vi "BME_DG_ResetCounters.vi"(7 "EventCounter(True)":bool=TRUE, 8 "error in (no error)":errorcluster, 9 "TileList(True)":bool=TRUE, 10 "ModuloCounter(True)":bool=TRUE, 11 "DG_Number":i32) -> (0 "error out":errorcluster, 3 "return code":i32)   [LabVIEW 2009, in "POLARIS BME DG.lvlib"]
uses:
  POLARIS BME DG.lvlib
  BME DLL/DelayGenerator.dll
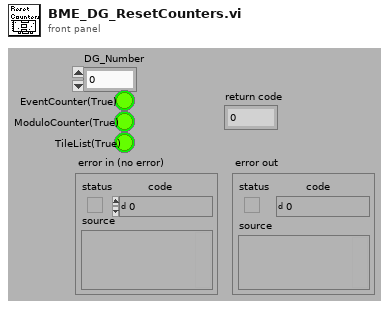
[diagram p1: front panel]
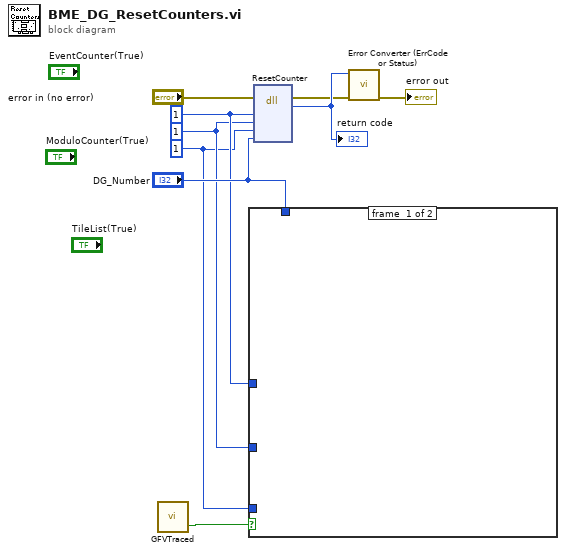
[diagram p0: block diagram]
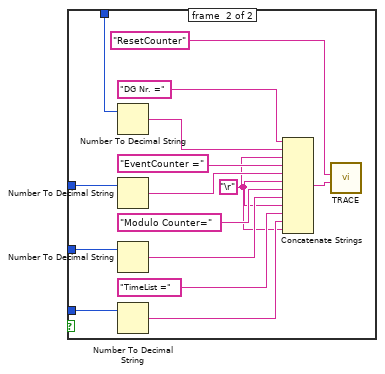
[diagram p2: hidden frame]
diagram:
  w1 = u32 1 ("bTimeList")
  w2 = u32 1 ("bTriggerCounter")
  w3 = u32 1 ("bEventCounter")
  n1 = call "GFVTraced.vi"() -> ("traced?"=w5:bool)  [unwired: 2 in]
  n2 = case shown="True" w5 {
    tunnel: w3 -> [_ w21]
    tunnel: w2 -> [_ w16]
    tunnel: "DG_Number" -> [_ w11]
    tunnel: w1 -> [_ w10]
    frame #0 {
    }
    frame #1 {
      w14 = "\r"
      n3 = Number To Decimal String(number=w11) -> (decimal integer string=w12:string)  [unwired: 1 in]
      n4 = Number To Decimal String(number=w21) -> (decimal integer string=w20:string)  [unwired: 1 in]
      n5 = Number To Decimal String(number=w16) -> (decimal integer string=w18:string)  [unwired: 1 in]
      n6 = Number To Decimal String(number=w10) -> (decimal integer string=w15:string)  [unwired: 1 in]
      n7 = Concatenate Strings("DG Nr. =", w12, w14, "EventCounter =", w20, w14, "Modulo Counter=", w18, w14, "TimeList =", w15, w14) -> (w22:string)
      n8 = call "TRACE.vi"("Parameter String"=w22, "Function"="ResetCounter") -> ()  [unwired: 10 in]
    }
  }
  n9 = dll-call lib="D:/CS Framework/LVSCC/LV2009/GPL/Projects/cs-framework/CSClass/CSPOLARIS/POLARIS BME DG/BME DLL/DelayGenerator.dll" fn="ResetCounter"(error in="error in (no error)", "bEventCounter"=w3, "bModuloCounter"=w2, "bTimeList"=w1, "dg_number"="DG_Number") -> (error out=w6:errorcluster, "return type"=w8:i32)  [unwired: 6 in, 1 out]
  "return code" <- w8
  n10 = call "Error Converter (ErrCode or Status).vi"("error in (no error)"=w6, "error code"=w8) -> ("error out"=→"error out":errorcluster)  [unwired: 9 in]
